vi "Get Analog Scaling.vi"(11 "Analog Configuration":T2) -> (3 "Analog Scaling":T1)   [LabVIEW 2013, in "PMU Recorder Light.lvlib" / "Statnett C37.118 DLL.lvclass"]
uses:
  Statnett C37.118 DLL.lvclass
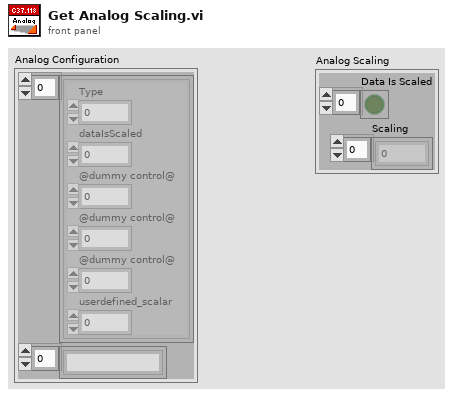
[diagram p1: front panel]
types:
  T1 = cluster{"Data Is Scaled":bool[], "Scaling":sgl[]}
  T2 = cluster{cluster{"Type":i32, "dataIsScaled":u8, "@dummy control@":i8, "@dummy control@":i8, "@dummy control@":i8, "userdefined_scalar":sgl}[], string[]}
  T3 = cluster{"Type":i32, "dataIsScaled":u8, "@dummy control@":i8, "@dummy control@":i8, "@dummy control@":i8, "userdefined_scalar":sgl}[]
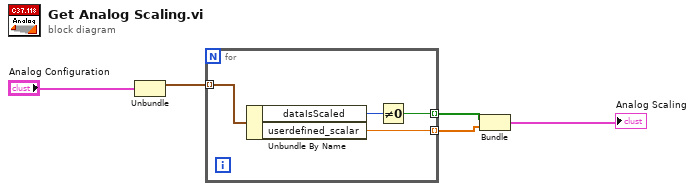
[diagram p0: block diagram]
diagram:
  n1 = Unbundle("Analog Configuration") -> (w5:T3)  [unwired: 1 out]
  n2 = for {
    tunnel: w5 -> [w9] mode=indexing
    tunnel: [w7] -> w3 mode=indexing
    tunnel: [w6] -> w2 mode=indexing
    n3 = Unbundle By Name(w9) -> ("dataIsScaled"=w8:u8, "userdefined_scalar"=w6:sgl)
    n4 = Not Equal To 0?(x=w8) -> (x != 0?=w7:bool)
  }
  n5 = Bundle(w3, w2) -> (→"Analog Scaling":cluster{bool[], sgl[]})  [unwired: 1 in]
